vi "Shake_table.vi"() -> ()   [LabVIEW 2015]
uses:
  <vilib>/MakerHub/LINX/Public/Peripherals/PWM/Set Duty Cycle 1 Chan.vi
  <vilib>/MakerHub/LINX/LMH-LINX.lvlib
panel:
  out "Speed":dbl(knob) scale=0.0..100.0
  out "percent":dbl
  out "random signal":dbl
  in  "white":u8
  in  "red":u8
  out "safe":bool
  out "danger":bool
  in  "LED brightness Pin":u8
  in  "Stop Button":bool
  in  "DC motor Pin":u8
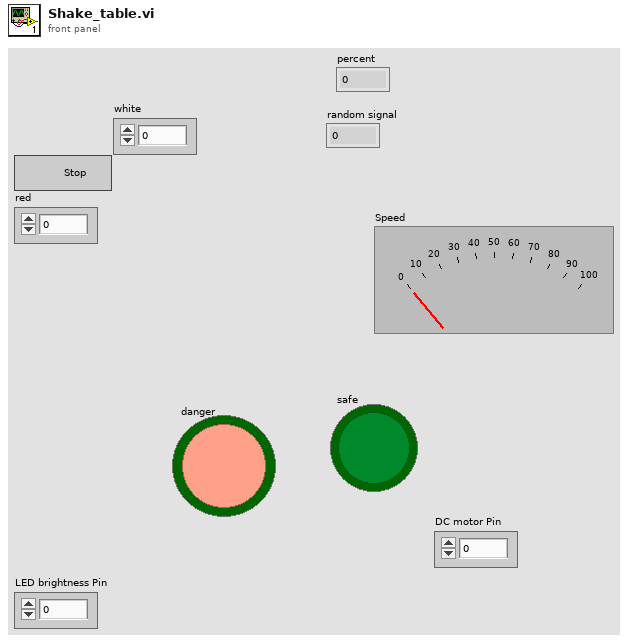
[diagram p1: front panel]
types:
  T1 = typedef "LMH-LINX.lvlib/LINX Ref.ctl" = cluster{"Platform":T2, "Interface":T3, "LINX Device Config":T4}
  T2 = typedef "LMH-LINX.lvlib/Platform.ctl" = enum16{"LINX", "myRIO"}
  T3 = typedef "LMH-LINX.lvlib/Interface.ctl" = enum16{"Serial", "TCP"}
  T4 = typedef "LMH-LINX.lvlib/Device.lvlib/LINX Device Config.ctl" = cluster{"Interface":T3, "COM Port":refnum<visa-resource-name>, "TCP Configuration":T5, "Device Family":u8, "Device ID":u8, "Device Name":string, "TCP Ref":refnum<k5>, "Channels":T6}
  T5 = typedef "LMH-LINX.lvlib/Device.lvlib/TCP Config.ctl" = cluster{"IP Address":string, "Port":u16}
  T6 = typedef "LMH-LINX.lvlib/Channels.ctl" = cluster{"DI":u8[], "DO":u8[], "AI":u8[], "AO":u8[], "PWM":u8[], "QE":u8[], "UART":u8[], "I2C 2":u8[], "SPI":u8[], "CAN":u8[], "Servo":u8[], "AI Ref (V)":dbl, "AO Ref (V)":dbl, "AO Resolution (Bits)":u8}
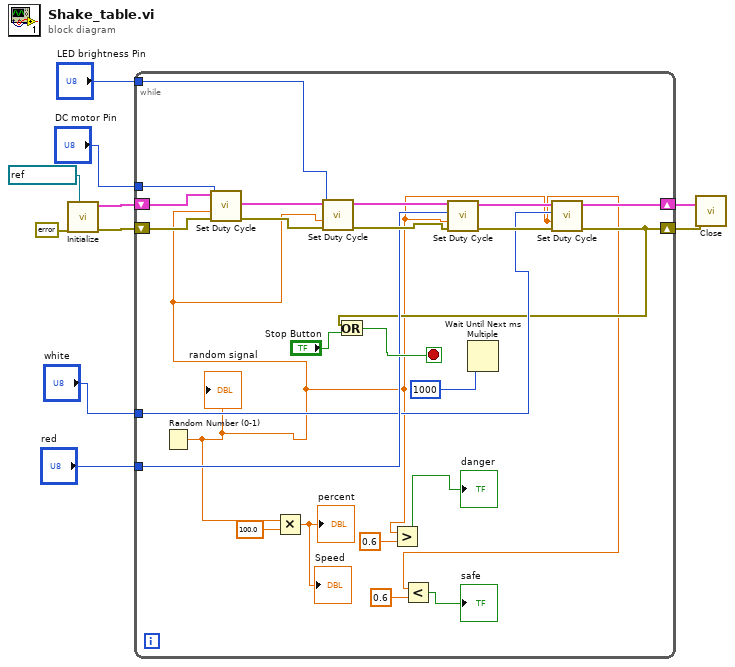
[diagram p0: block diagram]
diagram:
  n1 = call <vilib>:"Initialize.vi"("Serial Port"=refnum<visa-resource-name> "COM20", "Error In"=errorcluster {"status"=FALSE, "code"=0, "source"=""}) -> ("Error Out"=w8:errorcluster, "LINX Ref"=w10:T1)  [unwired: 7 in, 1 out]
  n2 = while {
    shift-right: [w16] -> w9
    shift-left: w10 -> [w34]
    shift-right: [w14] -> w7
    shift-left: w8 -> [w33]
    tunnel: "DC motor Pin" -> [w18]
    tunnel: "LED brightness Pin" -> [w28]
    tunnel: "red" -> [w20]
    tunnel: "white" -> [w15]
    stop <- w31 stop-if-true
    n3 = Random Number (0-1)() -> (number: 0 to 1=w13:dbl)
    "random signal" <- w13
    n4 = call-poly <vilib>:"Set Duty Cycle.vi"("Error In"=w33, "Duty Cycle (0-1)"=w13, "PWM Channel"=w18, "LINX Resource"=w34) -> ("Error Out"=w29:errorcluster, "LINX Resource"=w30:T1)  [unwired: 6 in]
    n5 = Multiply(x=w13, y=100.0) -> (x*y=→"percent" →"Speed":dbl)
    n6 = call-poly <vilib>:"Set Duty Cycle.vi"("Error In"=w29, "Duty Cycle (0-1)"=w13, "PWM Channel"=w28, "LINX Resource"=w30) -> ("Error Out"=w21:errorcluster, "LINX Resource"=w22:T1)  [unwired: 6 in]
    n7 = Greater?(x=w13, y=0.6) -> (0:→"danger":bool)
    n8 = Less?(x=w13, y=0.6) -> (x < y?=→"safe":bool)
    n9 = call-poly <vilib>:"Set Duty Cycle.vi"("Error In"=w21, "Duty Cycle (0-1)"=w13, "PWM Channel"=w20, "LINX Resource"=w22) -> ("Error Out"=w17:errorcluster, "LINX Resource"=w19:T1)  [unwired: 6 in]
    n10 = Wait Until Next ms Multiple(millisecond multiple=u32 1000) -> ()  [unwired: 1 out]
    n11 = call-poly <vilib>:"Set Duty Cycle.vi"("Error In"=w17, "Duty Cycle (0-1)"=w13, "PWM Channel"=w15, "LINX Resource"=w19) -> ("Error Out"=w14:errorcluster, "LINX Resource"=w16:T1)  [unwired: 6 in]
    n12 = Or(x=w14, y="Stop Button") -> (x .or. y?=w31:bool)
  }
  n13 = call <vilib>:"Close.vi"("Error In"=w7, "LINX Resource"=w9) -> ()  [unwired: 8 in, 2 out]
